vi "DoLoginUser.vi"(6 "error in (no error)":errorcluster, 8 "LoginName":string, 9 "Sequence Context In":refnum<k7>) -> (0 "error out":errorcluster, 3 "Sequence Context Out":refnum<k7>)   [LabVIEW 2021]
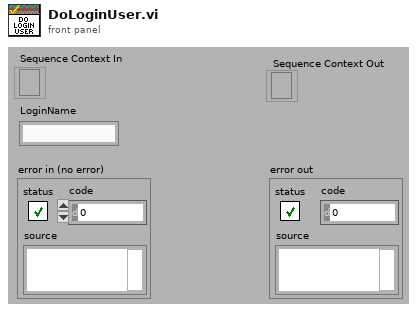
[diagram p1: front panel]
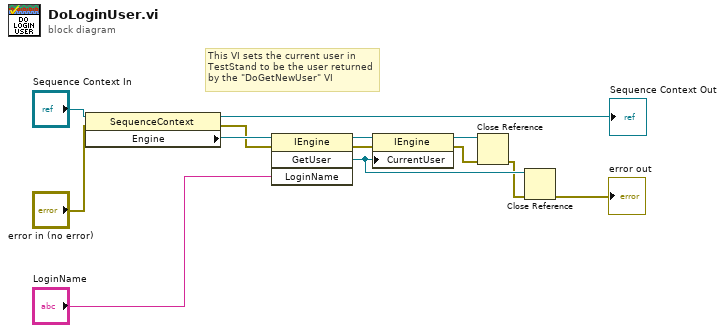
[diagram p0: block diagram]
diagram:
  # "This VI sets the current user in TestStand to be the user returned by the \"DoGetNewUser\" VI"
  n1 = property class="SequenceContext"(reference="Sequence Context In", error in="error in (no error)") -> (reference out=→"Sequence Context Out":refnum<k7>, error out=w5:errorcluster, "Engine"=w7:refnum<k7>)
  n2 = invoke class="IEngine" method="GetUser"(reference=w7, error in=w5, "LoginName"="LoginName") -> (reference out=w4:refnum<k7>, error out=w13:errorcluster, "GetUser"=w3:refnum<k7>)  [unwired: 1 in, 1 out]
  n3 = property class="IEngine"(reference=w4, error in=w13, "CurrentUser"=w3) -> (reference out=w10:refnum<k7>, error out=w9:errorcluster)
  n4 = Close Reference(reference=w10, error in (no error)=w9) -> (error out=w2:errorcluster)
  n5 = Close Reference(reference=w3, error in (no error)=w2) -> (error out=→"error out":errorcluster)
